vi "Destroy User Events.vi"(11 "UI Template in":refnum<class "StageController.lvclass">) -> (3 "UI Template out":refnum<class "StageController.lvclass">)   [LabVIEW 2020, in "StageController.lvlib" / "StageController.lvclass"]
uses:
  StageController.lvclass
  StageController.lvclass/StageController.ctl
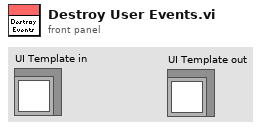
[diagram p1: front panel]
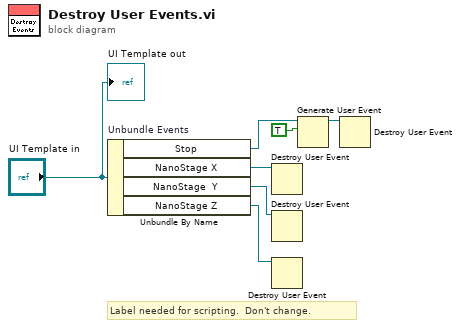
[diagram p0: block diagram]
diagram:
  # "Label needed for scripting.  Don't change."
  n1 = Unbundle By Name "Unbundle Events"("UI Template in") -> ("Stop"=w5:refnum<user-event>, "NanoStage X"=w3:refnum<user-event>, "NanoStage  Y"=w2:refnum<user-event>, "NanoStage Z"=w1:refnum<user-event>)
  n2 = Destroy User Event(user event=w3) -> ()  [unwired: 1 in, 1 out]
  n3 = Destroy User Event(user event=w2) -> ()  [unwired: 1 in, 1 out]
  n4 = Destroy User Event(user event=w1) -> ()  [unwired: 1 in, 1 out]
  n5 = Generate User Event(user event=w5, event data cluster=TRUE ("event data")) -> (user event out=w6:refnum<user-event>)  [unwired: 2 in, 1 out]
  n6 = Destroy User Event(user event=w6) -> ()  [unwired: 1 in, 1 out]
  "UI Template out" <- "UI Template in"
